vi "Single Command Execution.vi"() -> ()   [LabVIEW 2018]
doc: "Executes a single command on a remote SSH server. This is similar to connecting to executing a single command on a remote SSH server with a command line utility. This only works for executing a single command and reading its response. A new channel would have to be created to execute multiple channels or a SSH Shell with multiple write-read cycles would need to be implemented to execute multiple, sequential commands on a remote SSH server."
uses:
  Toolkit/Session/Support/Password Authentication.vi
  Toolkit/Channel/Support/Create from Session.vi
  Toolkit/Channel/Support/Destroy to Session.vi
  Toolkit/SSH/SSH.lvclass
  Toolkit/Session/Session.lvclass
  Toolkit/Channel/Channel.lvclass
panel:
  out "Response":string
  in  "Command":string="echo \"Hello World\""
  in  "Remote SSH Server":string
  in  "Password":string
  in  "Username":string
  # "Overview: Demonstrates executing a single command on a remote SSH server and reading back the response\nInstructions:\n1. Enter the IP address or host name of the remote SSH server. This can be a CompactRIO (cRIO) running the National Instruments Linux Real-Time (NI Linux RT) operating system with the Enable Secure Shell Server (sshd) checkbox checked. \n2. Enter a username. If using a cRIO with a default configuration, then the username is \"admin\".\n3. Enter a password for the username. If using a cRIO with a default configuration, then the password is blank (empty).\n4. Run this VI.\n5. Observe \"Hello World\" in the Response indicator.\n6. Change the command,\n7. Run this VI again."
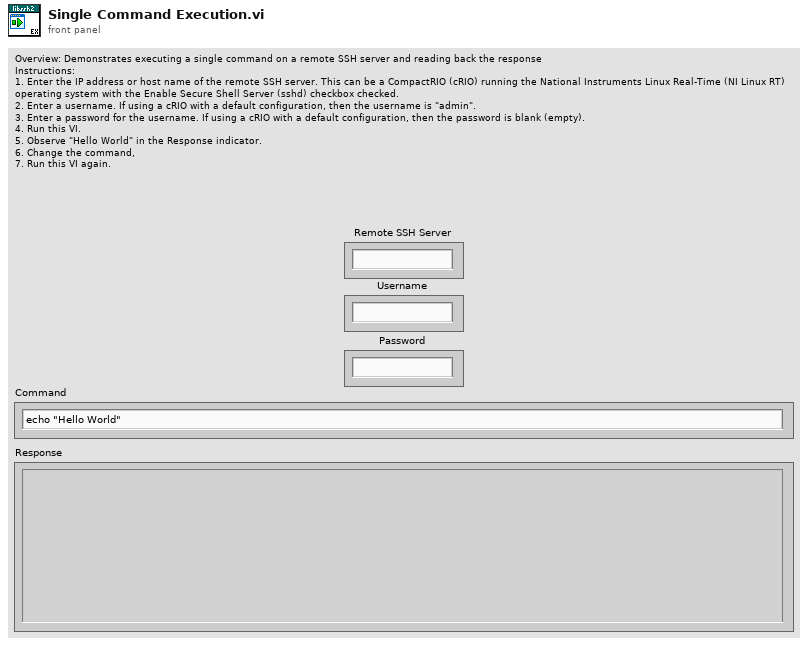
[diagram p1: front panel]
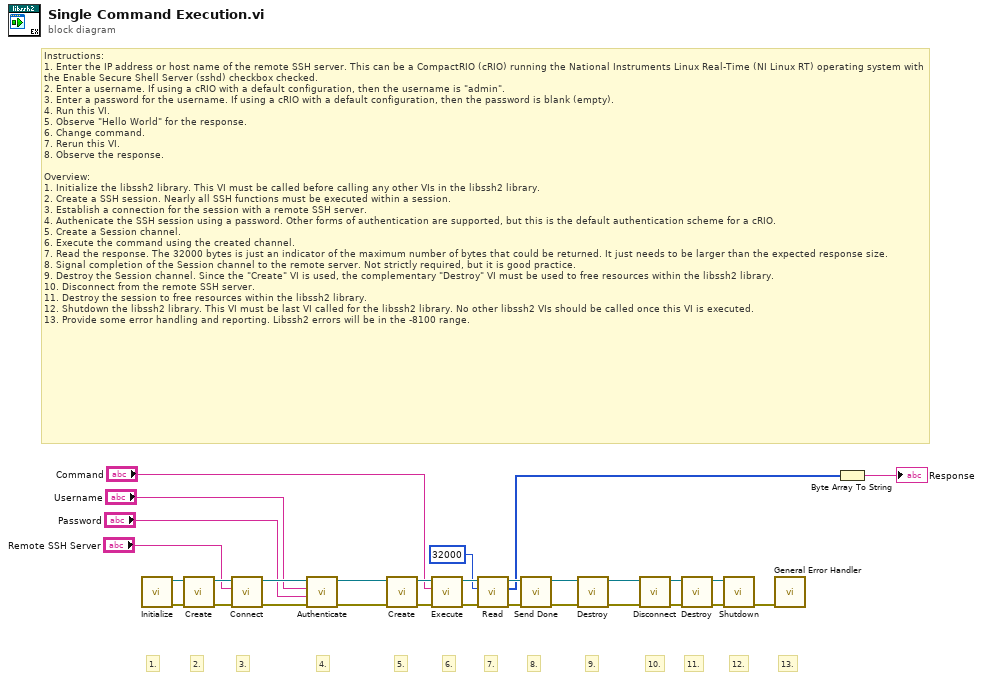
[diagram p0: block diagram]
diagram:
  # "13."
  # "12."
  # "11."
  # "10."
  # "9."
  # "8."
  # "7."
  # "6."
  # "5."
  # "4."
  # "3."
  # "2."
  # "1."
  # "Instructions:\n1. Enter the IP address or host name of the remote SSH server. This can be a CompactRIO (cRIO) running the National Instruments Linux Real-Time (NI Linux RT) operating system with the Enable Secure Shell Server (sshd) checkbox checked. \n2. Enter a username. If using a cRIO with a default configuration, then the username is \"admin\".\n3. Enter a password for the username. If using a cRIO with a default configuration, then the password is blank (empty).\n4. Run this VI.\n5. Observe \"Hello World\" for the response.\n6. Change command.\n7. Rerun this VI.\n8. Observe the response.\n\nOverview:\n1. Initialize the libssh2 library. This VI must be called before calling any other VIs in the libssh2 library.\n2. Create a SSH session. Nearly all SSH functions must be executed within a session.\n3. Establish a connection for the session with a remote SSH server.\n4. Authenicate the SSH session using a password. Other forms of authentication are supported, but this is the default authentication scheme for a cRIO. \n5. Create a Session channel.\n6. Execute the command using the created channel.\n7. Read the response. The 32000 bytes is just an indicator of the maximum number of bytes that could be returned. It just needs to be larger than the expected response size.\n8. Signal completion of the Session channel to the remote server. Not strictly required, but it is good practice.\n9. Destroy the Session channel. Since the \"Create\" VI is used, the complementary \"Destroy\" VI must be used to free resources within the libssh2 library.\n10. Disconnect from the remote SSH server.\n11. Destroy the session to free resources within the libssh2 library.\n12. Shutdown the libssh2 library. This VI must be last VI called for the libssh2 library. No other libssh2 VIs should be called once this VI is executed.\n13. Provide some error handling and reporting. Libssh2 errors will be in the -8100 range."
  n1 = call "Initialize.vi"() -> ("Error Out"=w29:errorcluster, "SSH"=w30:refnum<class "SSH.lvclass">)  [unwired: 10 in]
  n2 = call "Create.vi"("Error In"=w29, "SSH"=w30) -> ("Error Out"=w27:errorcluster, "Sesssion"=w28:refnum<class "Session.lvclass">)  [unwired: 8 in]
  n3 = call "Connect.vi"("Error In"=w27, "Address"="Remote SSH Server", "Session In"=w28) -> ("Error Out"=w25:errorcluster, "Sesssion Out"=w26:refnum<class "Session.lvclass">)  [unwired: 7 in]
  n4 = call-poly "Authenticate.vi"("Error In"=w25, "Password"="Password", "Username"="Username", "Session In"=w26) -> ("Error Out"=w23:errorcluster, "Sesssion Out"=w24:refnum<class "Session.lvclass">)  [unwired: 6 in]
  n5 = call-poly "Create.vi"("Error In"=w23, "Session"=w24) -> ("Error Out"=w21:errorcluster, "Channel"=w22:refnum<class "Channel.lvclass">)  [unwired: 8 in]
  n6 = call "Execute.vi"("Error In"=w21, "Command"="Command", "Channel In"=w22) -> ("Error Out"=w19:errorcluster, "Channel Out"=w20:refnum<class "Channel.lvclass">)  [unwired: 7 in]
  n7 = call "Read.vi"("Error In"=w19, "Max Data Length"=u64 32000, "Channel In"=w20) -> ("Error Out"=w17:errorcluster, "Data"=w7:u8[], "Channel Out"=w18:refnum<class "Channel.lvclass">)  [unwired: 6 in]
  n8 = call "Send Done.vi"("Error In"=w17, "Channel In"=w18) -> ("Error Out"=w15:errorcluster, "Channel Out"=w16:refnum<class "Channel.lvclass">)  [unwired: 8 in]
  n9 = call-poly "Destroy.vi"("Error In"=w15, "Channel"=w16) -> ("Error Out"=w13:errorcluster, "Session"=w14:refnum<class "Session.lvclass">)  [unwired: 8 in]
  n10 = call "Disconnect.vi"("Error In"=w13, "Session In"=w14) -> ("Error Out"=w11:errorcluster, "Sesssion Out"=w12:refnum<class "Session.lvclass">)  [unwired: 8 in]
  n11 = call "Destroy.vi"("Error In"=w11, "Session"=w12) -> ("Error Out"=w9:errorcluster, "SSH"=w10:refnum<class "SSH.lvclass">)  [unwired: 8 in]
  n12 = call "Shutdown.vi"("Error In"=w9, "SSH"=w10) -> ("Error Out"=w1:errorcluster)  [unwired: 9 in]
  n13 = call <vilib>:"General Error Handler.vi"("error in (no error)"=w1) -> ()  [unwired: 10 in, 5 out]
  n14 = Byte Array To String(unsigned byte array=w7) -> (string=→"Response":string)
